vi "programacio 7 tercer parcial.vi"() -> ()   [LabVIEW 2011]
panel:
  out "Array":T1(array[cluster]) {"Velocidad 3" scale=0.0..180.0; "Velocidad 2" scale=0.0..180.0; "Velocidad" scale=0.0..180.0}
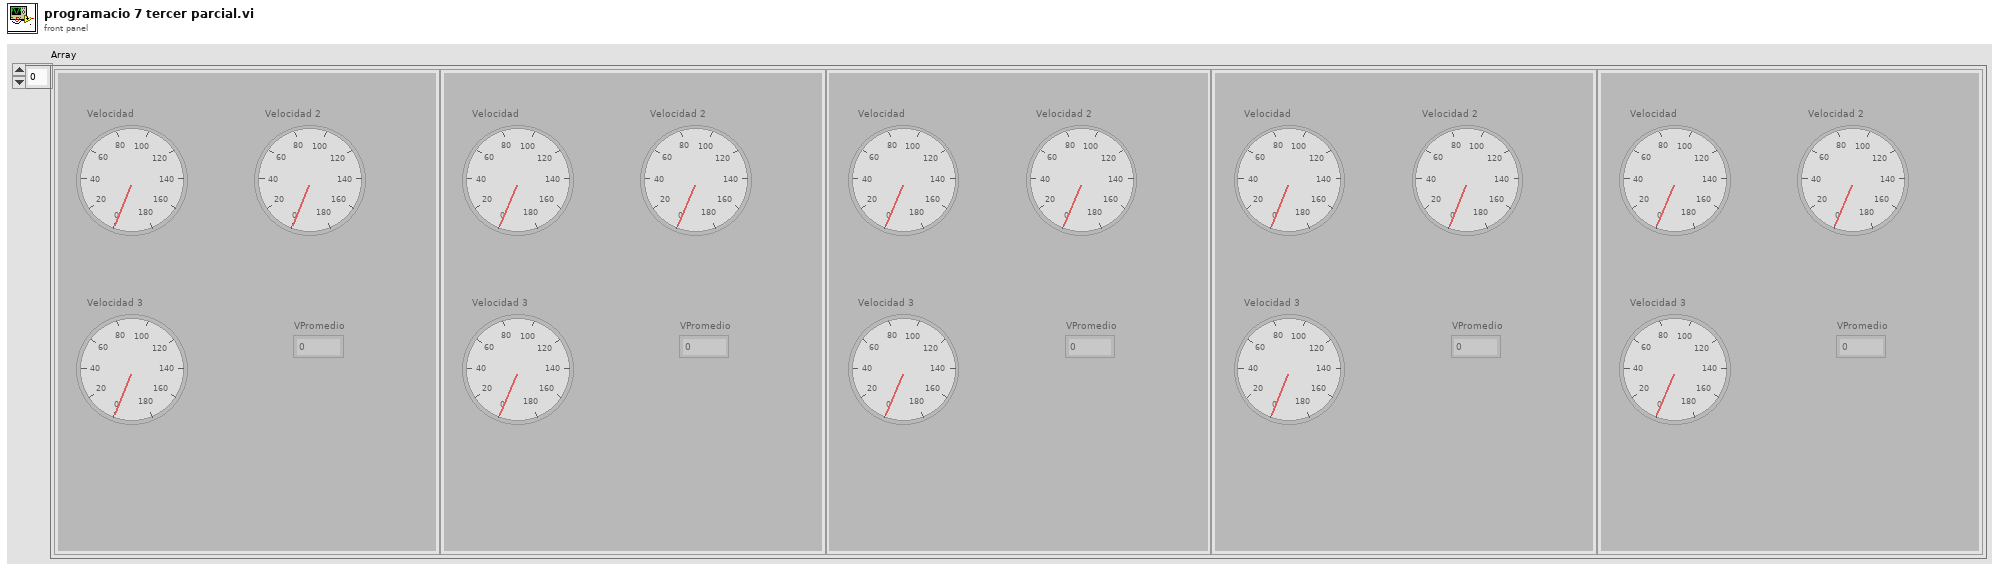
[diagram p1: front panel]
types:
  T1 = cluster{"Velocidad":i32, "Velocidad 2":i32, "Velocidad 3":i32, "VPromedio":dbl}[]
  T2 = enum16{"open", "replace", "create", "open or create", "replace or create", "replace or create with confirmation"}
  T3 = cluster{"Velocidad":i32, "Velocidad 2":i32, "Velocidad 3":i32, "VPromedio":dbl}
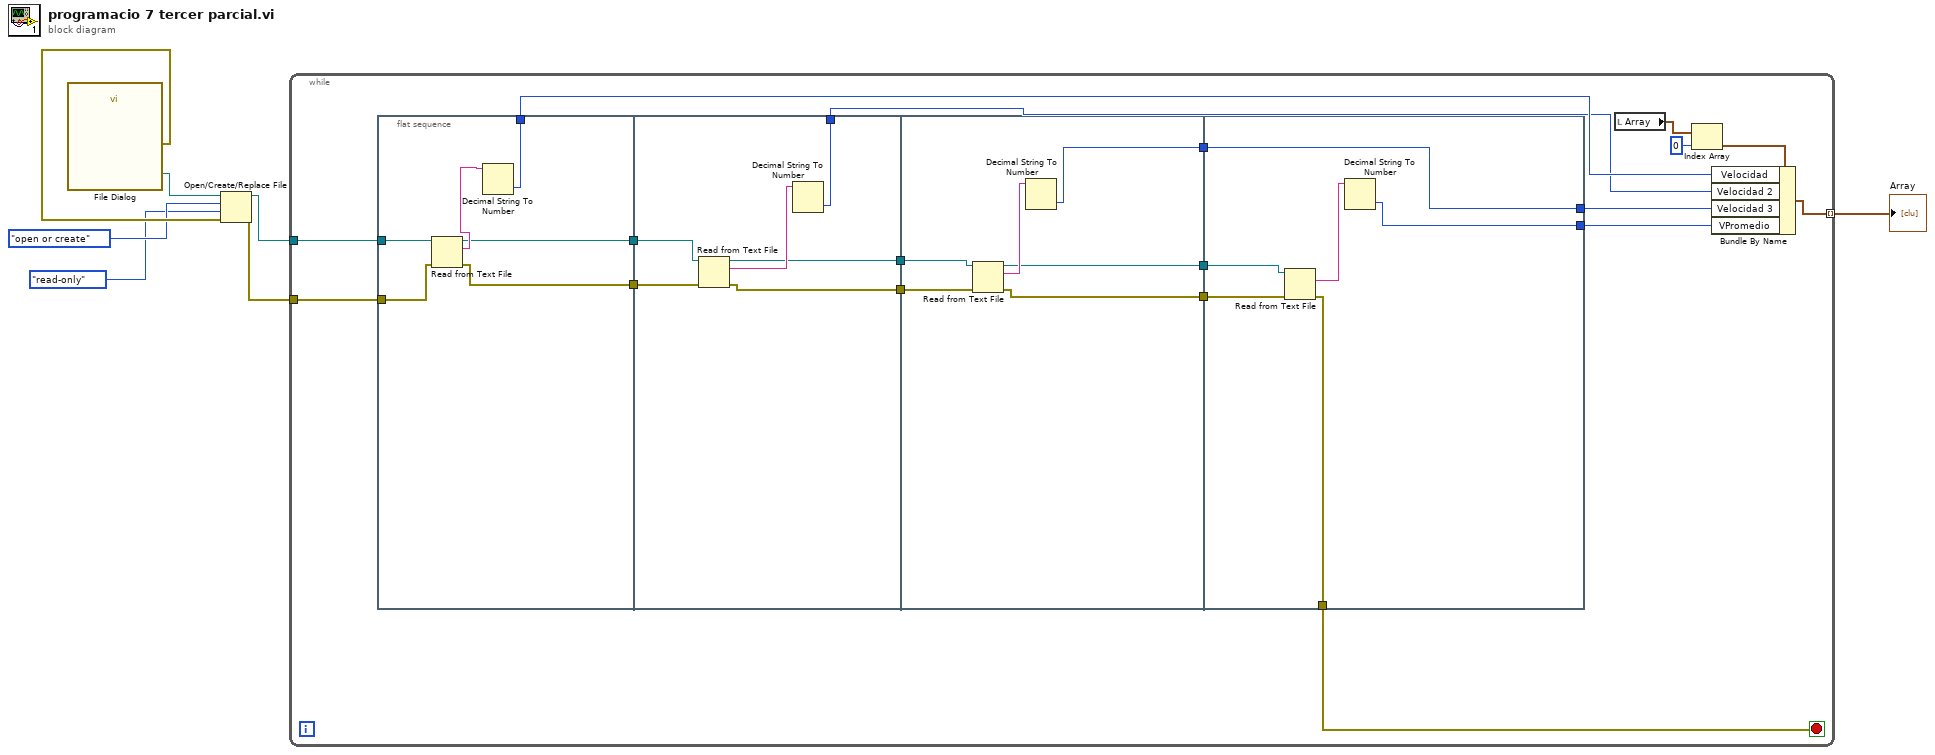
[diagram p0: block diagram]
diagram:
  n1 = call "File Dialog"() -> ("selected path"=w7:path, "error out"=w6:errorcluster)  [unwired: 12 in, 2 out]
  n2 = Open/Create/Replace File(file path (use dialog)=w7, error in=w6, operation (0:open)=T2."open or create", access (0:read/write)=enum16{"read/write", "read-only", "write-only"}."read-only") -> (refnum out=w3:refnum<file>, error out=w2:errorcluster)  [unwired: 2 in, 1 out]
  n3 = while {
    tunnel: w3 -> [w25]
    tunnel: w2 -> [w24]
    tunnel: [w9] -> w1 mode=indexing
    stop <- w8 stop-if-true
    n4 = flat-sequence {
      tunnel: w25 -> [w30]
      tunnel: w24 -> [w29]
      tunnel: [w28] -> w23
      tunnel: [w27] -> w22
      tunnel: [w26] -> w14
      tunnel: w23 -> [w37]
      tunnel: w22 -> [w36]
      tunnel: [w34] -> w21
      tunnel: [w33] -> w20
      tunnel: [w32] -> w13
      tunnel: w21 -> [w42]
      tunnel: w20 -> [w41]
      tunnel: [w40] -> w19
      tunnel: [w39] -> w18
      tunnel: [w38] -> w11
      tunnel: w19 -> [w48]
      tunnel: w18 -> [w47]
      tunnel: [w46] -> w12
      tunnel: w11 -> [w46]
      tunnel: [w45] -> w10
      tunnel: [w44] -> w8
      frame #0 {
        n5 = Read from Text File(file (use dialog)=w30, error in=w29) -> (refnum out=w27:refnum<file>, text=w31:string, error out=w28:errorcluster)  [unwired: 2 in, 1 out]
        n6 = Decimal String To Number(string=w31) -> (number=w26:i32)  [unwired: 2 in, 1 out]
      }
      frame #1 {
        n7 = Read from Text File(file (use dialog)=w36, error in=w37) -> (refnum out=w33:refnum<file>, text=w35:string, error out=w34:errorcluster)  [unwired: 2 in, 1 out]
        n8 = Decimal String To Number(string=w35) -> (number=w32:i32)  [unwired: 2 in, 1 out]
      }
      frame #2 {
        n9 = Read from Text File(file (use dialog)=w41, error in=w42) -> (refnum out=w39:refnum<file>, text=w43:string, error out=w40:errorcluster)  [unwired: 2 in, 1 out]
        n10 = Decimal String To Number(string=w43) -> (number=w38:i32)  [unwired: 2 in, 1 out]
      }
      frame #3 {
        n11 = Read from Text File(file (use dialog)=w47, error in=w48) -> (text=w49:string, error out=w44:errorcluster)  [unwired: 2 in, 2 out]
        n12 = Decimal String To Number(string=w49) -> (number=w45:i32)  [unwired: 2 in, 1 out]
      }
    }
    n13 = local read "Array"() -> (w17:T1)
    n14 = Index Array(array=w17, index=0) -> (element=w15:T3)
    n15 = Bundle By Name(cluster=w15, "Velocidad"=w14, "Velocidad 2"=w13, "Velocidad 3"=w12, "VPromedio"=w10) -> (w9:T3)
  }
  "Array" <- w1
